vi "CLI Build from Project Path.vi"() -> ()   [LabVIEW 2019, in "ProjectBuilder.lvlib"]
doc: "Run the 'Load and Build'-vi using the given CLI arguments.\n\nRequired arguments:\nProject: \"Project=[path to project]\" - Path to the project file to act on.\n\nOptional arguments:\nQuit: \"Quit\" - Optional. Terminate LabVIEW after finishing the build actions.\nReport: \"Report=[path to report folder] - Optional\nConfig: \"Config=[path to override config file] - Optional\nBuilderName: \"BuilderName=[simple class name for the builder class to use] - Optional\nBuilderData: \"BuilderData=[string data] - Optional. Data will be used in the Populate.vi."
uses:
  ProjectBuilder.lvlib
  PPL/HDH.ClassLoader.lvlibp
  ca36580e-110a-4bd8-b9a5-6617d43ed2ad.vi
  <vilib>/ErrorRing/Error Ring.xnode
  Class/Project Builder/Project Builder.lvclass
  <vilib>/Utility/error.llb/Error Cluster From Error Code.vi
panel:
  out "value out":errorcluster
  out "Quit after execution?":bool
  out "Valid project?":bool
  out "Project path":path
  # "Running 'Build Project' on:"
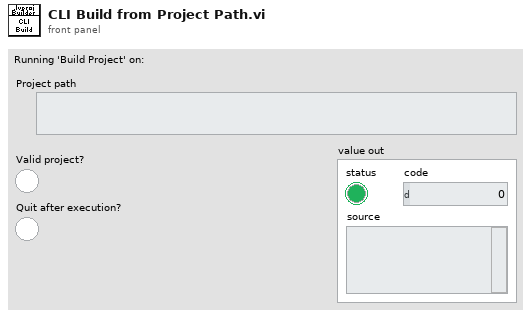
[diagram p1: front panel]
types:
  T1 = cluster{"Project path":path, "Report Folder":path, "Quit?":bool, "Builder Name":string, "Builder Data":string, "Config Override":path}
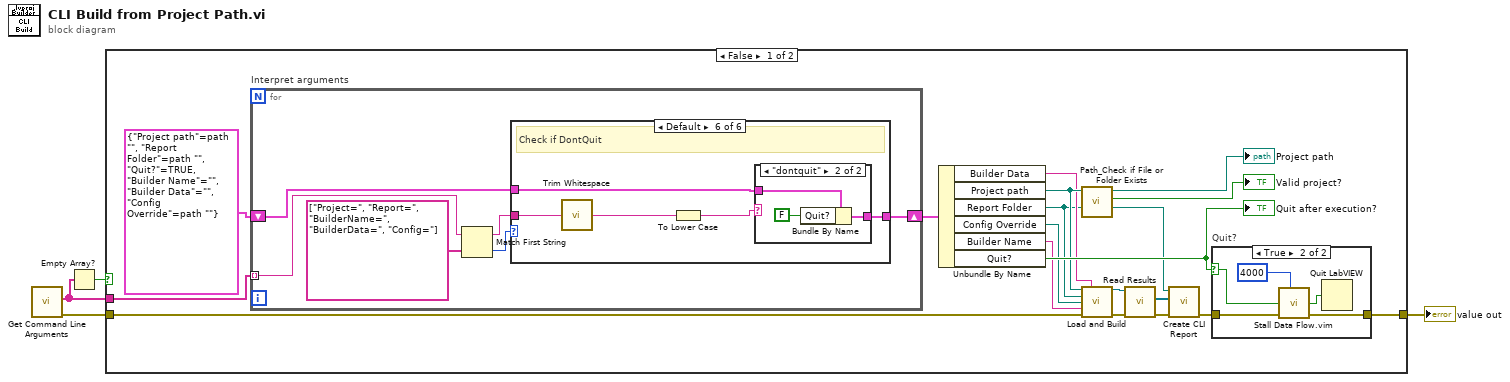
[diagram p0: block diagram]
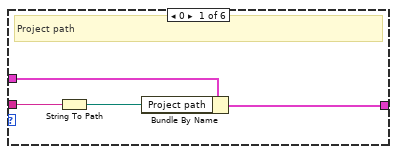
[diagram p3: hidden frame]
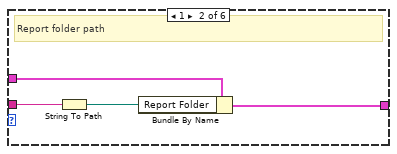
[diagram p4: hidden frame]
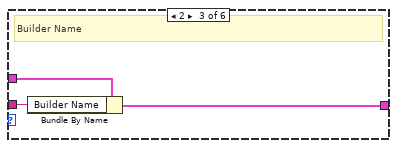
[diagram p5: hidden frame]
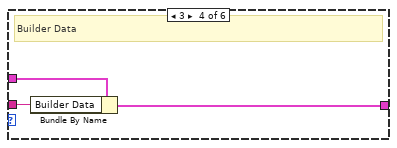
[diagram p6: hidden frame]
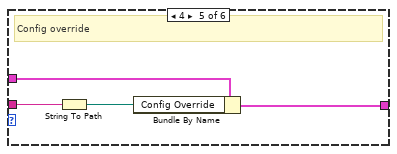
[diagram p7: hidden frame]
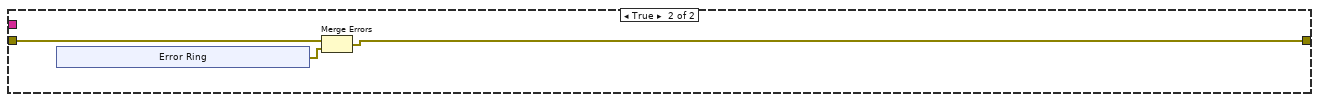
[diagram p9: hidden frame]
diagram:
  n1 = call <vilib>:"Get Command Line Arguments.vi"() -> ("error out"=w4:errorcluster, "arguments"=w3:string[])  [unwired: 9 in, 1 out]
  n2 = Empty Array?(array=w3) -> (empty?=w2:bool)
  n3 = case shown="False" w2 {
    tunnel: w4 -> [w6 w63]
    tunnel: w3 -> [w22 _]
    tunnel: [w13 w62] -> w1
    frame False {
      n4 = for "Interpret arguments" {
        tunnel: w22 -> [w32] mode=indexing
        shift-right: [w28] -> w20
        shift-left: T1 {"Project path"=path "", "Report Folder"=path "", "Quit?"=TRUE, "Builder Name"="", "Builder Data"="", "Config Override"=path ""} -> [w29]
        n5 = Match First String(2:string[] ["Project=", "Report=", "BuilderName=", "BuilderData=", "Config="] ("string array"), 3:w32) -> (0:w30:i32, 1:w31:string)
        n6 = case shown="Default" w30 {
          tunnel: w31 -> [w36 w41 w43 w46 w50 w55]
          tunnel: w29 -> [w34 w40 w44 w47 w48 w53]
          tunnel: [w35 w38 w42 w45 w49 w54] -> w28
          frame 0 {
            # "Project path"
            n7 = String To Path(string=w36) -> (path=w37:path)
            n8 = Bundle By Name(cluster=w34, "Project path"=w37) -> (w35:T1)
          }
          frame 1 {
            # "Report folder path"
            n9 = String To Path(string=w41) -> (path=w39:path)
            n10 = Bundle By Name(cluster=w40, "Report Folder"=w39) -> (w38:T1)
          }
          frame 2 {
            # "Builder Name"
            n11 = Bundle By Name(cluster=w44, "Builder Name"=w43) -> (w42:T1)
          }
          frame 3 {
            # "Builder Data"
            n12 = Bundle By Name(cluster=w47, "Builder Data"=w46) -> (w45:T1)
          }
          frame 4 {
            # "Config override"
            n13 = String To Path(string=w50) -> (path=w51:path)
            n14 = Bundle By Name(cluster=w48, "Config Override"=w51) -> (w49:T1)
          }
          frame Default {
            # "Check if DontQuit"
            n15 = call <vilib>:"Trim Whitespace.vi"("string"=w55) -> ("trimmed string"=w56:string)  [unwired: 1 in]
            n16 = To Lower Case(string=w56) -> (all lower case string=w52:string)
            n17 = case shown="\"dontquit\"" w52 {
              tunnel: [w57 w59] -> w54
              tunnel: w53 -> [w57 w60]
              frame Default {
              }
              frame "dontquit" {
                n18 = Bundle By Name(cluster=w60, "Quit?"=FALSE) -> (w59:T1)
              }
            }
          }
        }
      }
      n19 = Unbundle By Name(w20) -> ("Builder Data"=w15:string, "Project path"=w16:path, "Report Folder"=w7:path, "Config Override"=w5:path, "Builder Name"=w14:string, "Quit?"=w19:bool)
      "Quit after execution?" <- w19
      n20 = call "Path_Check if File or Folder Exists.vi"("File or Folder Path in"=w16) -> ("File or Folder Found?"=→"Valid project?":bool, "File or Folder Path dub"=→"Project path":path)  [unwired: 9 in]
      n21 = call "Load and Build.vi"("Project Path"=w16, "Data String (\"\")"=w15, "Report Folder"=w7, "Build Config Override"=w5, "Project Build Class Name (Empty = \"Project Builder\")"=w14, "error in (no error)"=w6) -> ("Project Builder out"=w12:refnum<class "Project Builder.lvclass">, "error out"=w11:errorcluster)  [unwired: 7 in, 1 out]
      n22 = call "Read Results.vi"("error in (no error)"=w11, "Project Builder in"=w12) -> ("error out"=w10:errorcluster, "Results"=w8:refnum<class "Report Data.lvclass">[])  [unwired: 7 in, 1 out]
      n23 = call "Create CLI Report.vi"("error in (no error)"=w10, "Results"=w8, "Report Folder"=w7) -> ("error dub"=w9:errorcluster)  [unwired: 8 in]
      n24 = case "Quit?" shown="True" w19 {
        selector: w19 -> [_ w26]
        tunnel: w9 -> [w23 w27]
        tunnel: [w23 w27] -> w13
        frame False {
        }
        frame True {
          n25 = call "Stall Data Flow.vim"("value in"=w26, "milliseconds to wait"=u32 4000) -> ("value out"=w24:bool)  [unwired: 1 out]
          n26 = Quit LabVIEW(quit? (T)=w24) -> ()
        }
      }
    }
    frame True {
      n27 = xnode "Error Ring"() -> ("error out"=w61:errorcluster)
      n28 = Merge Errors(w63, w61) -> (w62:errorcluster)
    }
  }
  "value out" <- w1
